vi "CCE RRMA P01 SubVI03.vi"(5 "d":dbl, 7 "f":dbl, 9 "xi":u32, 10 "xd":u32, 11 "array":u32[][](array[numeric])) -> (2 "X":i32, 3 "Z":i32)   [LabVIEW 2020]
doc: "Ceballos Conde Emanuel Rodríguez Ramírez Miguel Ángel 4MV6 Sistemas de visión artificial 2022/1\nEste vi realiza el calculo de la distancia en X y Z utilizando los centroides obtenidos de las capturas des sisitema de vision estereoscopica, los centroides ingresados deben de ser respecto al origen de la imagen ya que el vi realiza la conversion de estos a un centriode respecto al centro de la imagen"
panel:
  out "xcd":dbl
  out "xci":dbl
  in  "yi":u32
  in  "yd":u32
  # "Ceballos Conde Emanuel\nRodríguez Ramírez Miguel Ángel\n4MV6\nSistemas de visión artificial\n2022/1"
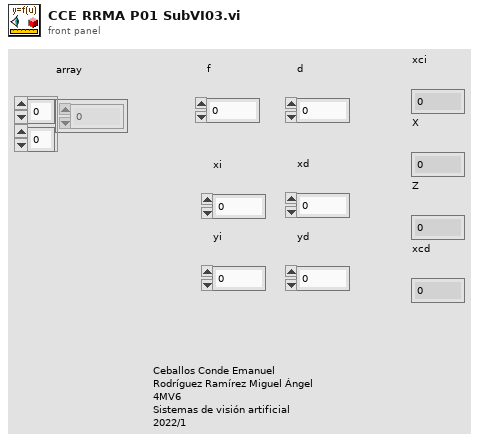
[diagram p1: front panel]
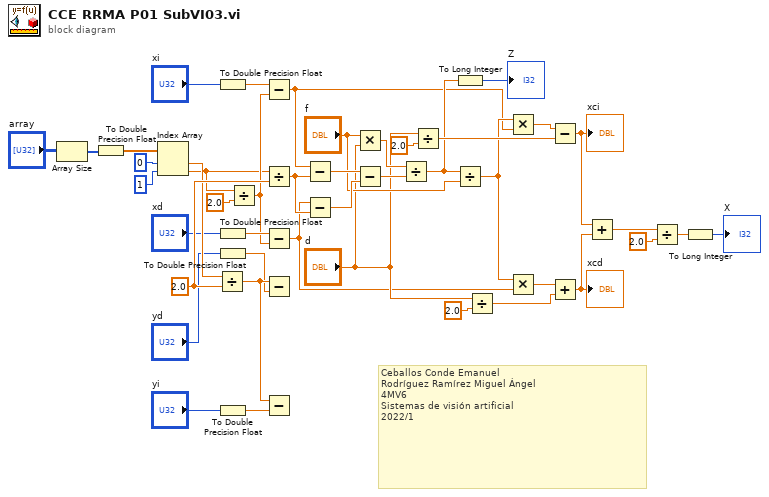
[diagram p0: block diagram]
diagram:
  w37 = 2.0 ("y")
  # "Ceballos Conde Emanuel\nRodríguez Ramírez Miguel Ángel\n4MV6\nSistemas de visión artificial\n2022/1"
  n1 = Array Size(array="array") -> (size(s)=w42:i32[])
  n2 = To Double Precision Float(number=w42) -> (double precision float=w38:dbl[])
  n3 = Index Array(array=w38, index #1=0 ("index"), index #2=1 ("index")) -> (element #1=w36:dbl, element #2=w1:dbl)
  n4 = Divide(x=w36, y=w37) -> (x/y=w32:dbl)
  n5 = To Double Precision Float(number="xi") -> (double precision float=w23:dbl)
  n6 = To Double Precision Float(number="xd") -> (double precision float=w13:dbl)
  n7 = To Double Precision Float(number="yd") -> (double precision float=w26:dbl)
  n8 = To Double Precision Float(number="yi") -> (double precision float=w25:dbl)
  n9 = Divide(x=w1, y=2.0) -> (x/y=w3:dbl)
  n10 = Subtract(x=w23, y=w3) -> (x-y=w7:dbl)
  n11 = Divide(x=w1, y=w37) -> (x/y=w31:dbl)
  n12 = Subtract(x=w13, y=w3) -> (x-y=w6:dbl)
  n13 = Subtract(x=w32, y=w26) -> ()  [unwired: 1 out]
  n14 = Subtract(x=w32, y=w25) -> ()  [unwired: 1 out]
  n15 = Subtract(x=w7, y=w31) -> (x-y=w30:dbl)
  n16 = Subtract(x=w6, y=w31) -> (x-y=w29:dbl)
  n17 = Multiply(x="f", y="d") -> (x*y=w28:dbl)
  n18 = Subtract(x=w30, y=w29) -> (x-y=w27:dbl)
  n19 = Divide(x=w28, y=w27) -> (x/y=w16:dbl)
  n20 = Divide(x="d", y=2.0) -> (x/y=w20:dbl)
  n21 = To Long Integer(number=w16) -> (32bit integer=→"Z":i32)
  n22 = Divide(x=w16, y="f") -> (x/y=w14:dbl)
  n23 = Divide(x="d", y=2.0) -> (x/y=w18:dbl)
  n24 = Multiply(x=w14, y=w7) -> (x*y=w22:dbl)
  n25 = Multiply(x=w14, y=w6) -> (x*y=w15:dbl)
  n26 = Subtract(x=w22, y=w20) -> (x-y=w11:dbl)
  "xci" <- w11
  n27 = Add(x=w15, y=w18) -> (x+y=w10:dbl)
  "xcd" <- w10
  n28 = Add(x=w11, y=w10) -> (x+y=w9:dbl)
  n29 = Divide(x=w9, y=2.0) -> (x/y=w8:dbl)
  n30 = To Long Integer(number=w8) -> (32bit integer=→"X":i32)
